vi "lab2ChannelsToImage.vi"(0 "imgWidth":i32, 1 "imgHeight":i32, 5 "blueChannel":u8[](array[numeric]), 6 "greenChannel":u8[](array[numeric]), 7 "redChannel":u8[](array[numeric]), 8 "channel4":u8[](array[numeric])) -> (2 "image data":T1)   [LabVIEW 2016]
uses:
  <vilib>/picture/picture.llb/imagedata.ctl
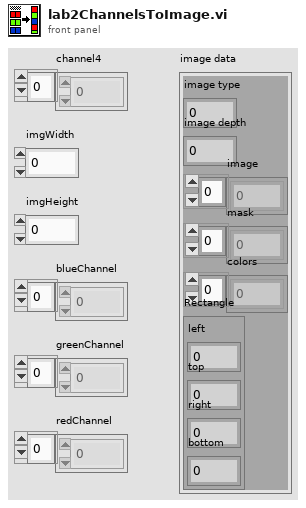
[diagram p1: front panel]
types:
  T1 = typedef "imagedata.ctl" = cluster{"image type":i32, "image depth":i32, "image":u8[], "mask":u8[], "colors":u32[], "Rectangle":cluster{"left":i16, "top":i16, "right":i16, "bottom":i16}}
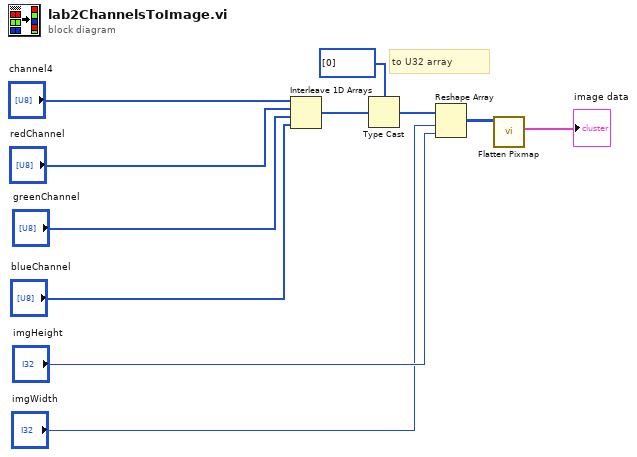
[diagram p0: block diagram]
diagram:
  # "to U32 array"
  n1 = Interleave 1D Arrays("channel4", "redChannel", "greenChannel", "blueChannel") -> (w4:u8[])
  n2 = Type Cast(type=u32[] [0], x=w4) -> (*(type *) &x=w5:u32[])
  n3 = Reshape Array(w5, "imgWidth", "imgHeight") -> (w2:u32[][])
  n4 = call <vilib>:"Flatten Pixmap.vi"("24-bit pixmap"=w2) -> ("image data"=→"image data":T1)  [unwired: 10 in]
